vi "Get VI Reference.vi"(8 "error in (no error)":errorcluster, 11 "VI Reference Control in":refnum<class "VI Reference Control.lvclass">) -> (0 "error out":errorcluster, 2 "VI Ref":refnum<vi>, 3 "VI Reference Control out":refnum<class "VI Reference Control.lvclass">)   [LabVIEW 2016, in "VI Reference Control.lvclass"]
uses:
  VI Reference Control.lvclass
  VI Reference Control.lvclass/VI Reference Control.ctl
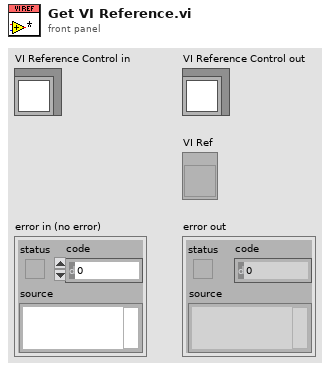
[diagram p1: front panel]
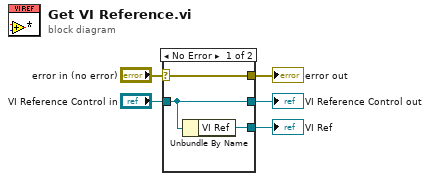
[diagram p0: block diagram]
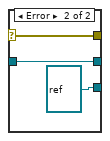
[diagram p2: hidden frame]
diagram:
  n1 = case shown="No Error" "error in (no error)" {
    selector: "error in (no error)" -> [w8 w11]
    tunnel: [w8 w11] -> w4
    tunnel: [w7 w10] -> w2
    tunnel: "VI Reference Control in" -> [w7 w10]
    tunnel: [w6 refnum<vi> refnum ("VI Ref")] -> w1
    frame No Error {
      n2 = Unbundle By Name(w7) -> ("VI Ref"=w6:refnum<vi>)
    }
    frame Error {
    }
  }
  "error out" <- w4
  "VI Reference Control out" <- w2
  "VI Ref" <- w1
